vi "Create Bus ShapeRef.vi"(8 "error in (no error)":errorcluster, 11 "Picture in":refnum<vi>) -> (0 "error out":errorcluster, 3 "Data Value Reference out":refnum<data-value>)   [LabVIEW 2015]
uses:
  <vilib>/LIEF/Forms/Shape/Shape.lvclass
  Bus/Bus.lvclass
  <vilib>/LIEF/Forms/Shape/Shape.lvclass/Shape.ctl
  <vilib>/LIEF/Forms/Shape/Write Color.vi
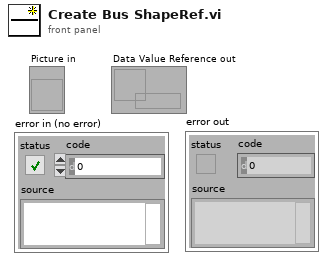
[diagram p1: front panel]
types:
  T1 = typedef "LVBoundsTypeDef.ctl" = cluster{"Width":u32, "Height":u32}
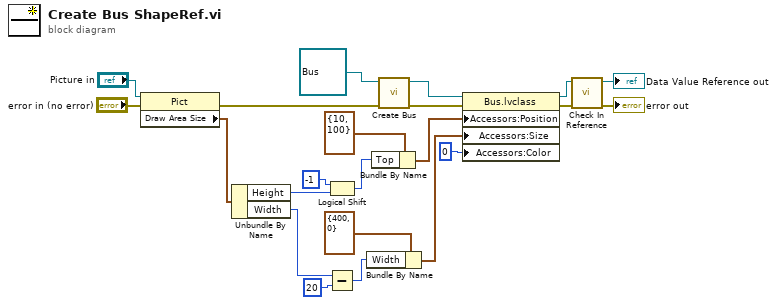
[diagram p0: block diagram]
diagram:
  n1 = property class="Pict"(reference="Picture in", error in="error in (no error)") -> (error out=w2:errorcluster, "Draw Area Size"=w11:T1)  [unwired: 1 out]
  n2 = Unbundle By Name(w11) -> ("Height"=w16:u32, "Width"=w12:u32)
  n3 = Logical Shift(y=i16 -1, x=w16) -> (x << y=w19:u32)
  n4 = Subtract(x=w12, y=u32 20) -> (x-y=w15:u32)
  n5 = Bundle By Name(cluster=cluster{"Width":i32, "Height":i32} {"Width"=400, "Height"=0} ("Size"), "Width"=w15) -> (w21:cluster{"Width":i32, "Height":i32})
  n6 = Bundle By Name(cluster=cluster{"Left":i32, "Top":i32} {"Left"=10, "Top"=100} ("Position"), "Top"=w19) -> (w20:cluster{"Left":i32, "Top":i32})
  n7 = call "Create Bus.vi"("error in (no error)"=w2, "Bus in"=refnum<class "Bus.lvclass"> refnum ("Bus.lvclass")) -> ("error out"=w1:errorcluster, "Bus out"=w6:refnum<class "Bus.lvclass">)  [unwired: 8 in]
  n8 = property class="Bus.lvclass"(reference=w6, error in=w1, "Accessors:Position"=w20, "Accessors:Size"=w21, "Accessors:Color"=u32 0 ("Color")) -> (reference out=w7:refnum<class "Bus.lvclass">, error out=w8:errorcluster)
  n9 = call <vilib>:"Check In Reference.vi"("error in (no error)"=w8, "Shape in"=w7) -> ("error out"=→"error out":errorcluster, "Shape Reference"=→"Data Value Reference out":refnum<data-value>)  [unwired: 8 in]
